vi "WPI_Gyro_ADXRS453_ReadRegister.vi"(8 "error in (no error)":errorcluster, 10 "ADXRS453 Register":T3 items=["Rate"=0, "Tem"=2, "LoCST"=4, "HiCST"=6, "Quad"=8, "Fault"=10, "PID"=12, "SN High"=14, "SN Low"=16], 11 "SPIDevRef in":T1) -> (0 "error out":errorcluster, 2 "Register Value":u16, 3 "SPIDevRef out":T1)   [LabVIEW 2015, in "SimpleGyro.lvlib"]
uses:
  SimpleGyro.lvlib
  <vilib>/Rock Robotics/WPI/SPI/WPI_SPIDevRef.ctl
  <vilib>/Rock Robotics/SystemInterfaces/spilib/spi_bus.ctl
  WPI_Gyro_ADXRS453_Registers.ctl
  WPI_Gyro_ADXRS453_Commands.ctl
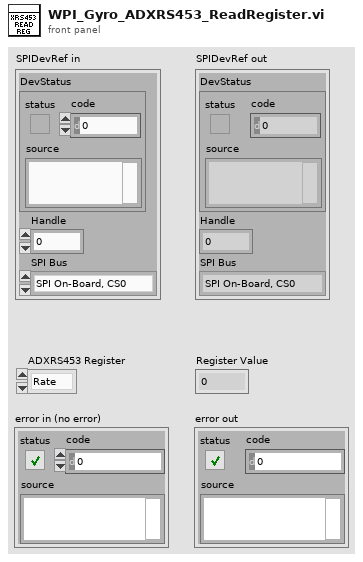
[diagram p1: front panel]
types:
  T1 = typedef "WPI_SPIDevRef.ctl" = cluster{"DevStatus":errorcluster, "Handle":i32, "SPI Bus":T2}
  T2 = typedef "spi_bus.ctl" = enum16{"SPI On-Board, CS0", "SPI On-Board, CS1", "SPI On-Board, CS2", "SPI On-Board, CS3", "SPI MXP", "Invalid"}
  T3 = typedef "SimpleGyro.lvlib/WPI_Gyro_ADXRS453_Registers.ctl" = u16
  T4 = typedef "SimpleGyro.lvlib/WPI_Gyro_ADXRS453_Commands.ctl" = u8
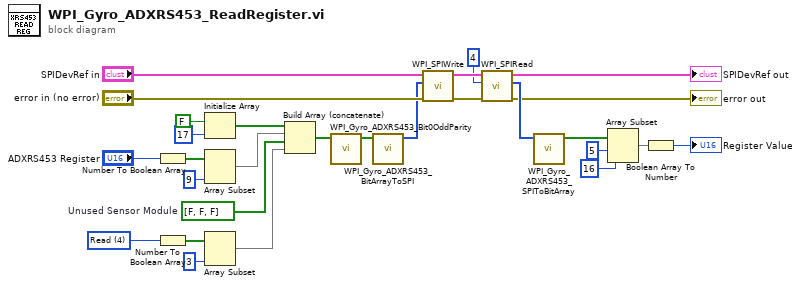
[diagram p0: block diagram]
diagram:
  w27 = bool[] [FALSE, FALSE, FALSE]  # Unused Sensor Module
  w4 = T4 4 items=["Read"=4, "Write"=2, "Sensor Data"=1]
  n1 = Number To Boolean Array(number="ADXRS453 Register") -> (Boolean array=w8:bool[])
  n2 = Number To Boolean Array(number=w4) -> (Boolean array=w5:bool[])
  n3 = Initialize Array(FALSE, 17 ("dimension size")) -> (w13:bool[])
  n4 = Array Subset(array=w8, length=9) -> (w14:bool[])  [unwired: 1 in]
  n5 = Array Subset(array=w5, length=3) -> (w15:bool[])  [unwired: 1 in]
  n6 = Build Array (concatenate)(w13, w14, w27, w15) -> (w12:bool[])
  n7 = call "WPI_Gyro_ADXRS453_Bit0OddParity.vi"("Array in"=w12) -> ("Array out"=w16:bool[])  [unwired: 10 in]
  n8 = call "WPI_Gyro_ADXRS453_BitArrayToSPI.vi"("32-bit Array in"=w16) -> ("SPI Byte Array (MSB first)"=w17:u8[])  [unwired: 10 in]
  n9 = call <vilib>:"WPI_SPIWrite.vi"("error in (no error)"="error in (no error)", "Data To Send"=w17, "SPIDevRef"="SPIDevRef in") -> ("error out"=w25:errorcluster, "SPIDevRef"=w3:T1)  [unwired: 7 out]
  n10 = call <vilib>:"WPI_SPIRead.vi"("error in (no error)"=w25, "Num to Read"=4, "SPIDevRef"=w3) -> ("error out"=→"error out":errorcluster, "Received Data"=w19:u8[], "SPIDevRef"=→"SPIDevRef out":T1)  [unwired: 6 in]
  n11 = call "WPI_Gyro_ADXRS453_SPIToBitArray.vi"("SPI Byte Array (MSB first)"=w19) -> ("32-bit Boolean array"=w20:bool[])  [unwired: 10 in]
  n12 = Array Subset(array=w20, index=5, length=16) -> (w23:bool[])
  n13 = Boolean Array To Number(Boolean array=w23) -> (number=→"Register Value":u16)
